vi "QBuf.vi"(3 "error in (no error)":errorcluster, 4 "pBufferHandle":i64, 5 "nInputHandle":u64) -> (0 "error out":errorcluster, 1 "GX_STATUS":i32, 2 "nOutputHandle":u64)   [LabVIEW 2016, in "GxLVLib.lvlib"]
uses:
  GxLVLib.lvlib
  GxIAPI.dll
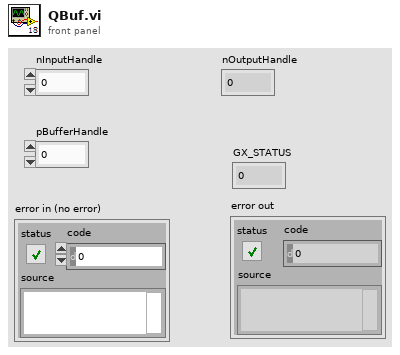
[diagram p1: front panel]
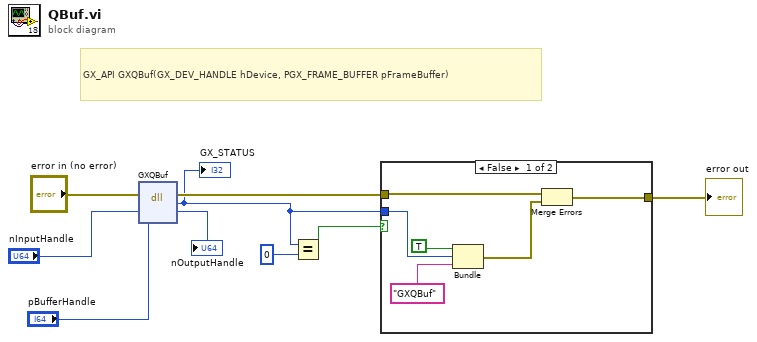
[diagram p0: block diagram]
diagram:
  # "GX_API GXQBuf(GX_DEV_HANDLE hDevice, PGX_FRAME_BUFFER pFrameBuffer)"
  n1 = dll-call lib="GxIAPI.dll" fn="GXQBuf"(error in="error in (no error)", "phDevice"="nInputHandle", "pBufferHandle"="pBufferHandle") -> (error out=w6:errorcluster, "GX_STATUS"=w3:i32, "phDevice"=→"nOutputHandle":i64)  [unwired: 3 in, 1 out]
  "GX_STATUS" <- w3
  n2 = Equal?(x=w3, y=0) -> (x = y?=w7:bool)
  n3 = case shown="False" w7 {
    tunnel: w6 -> [w15 w16]
    tunnel: [w14 w16] -> w5
    tunnel: w3 -> [w12 _]
    frame False {
      n4 = Bundle(TRUE, "GX_STATUS"=w12, "GXQBuf") -> (w13:cluster{bool, "GX_STATUS":i32, string})  [unwired: 1 in]
      n5 = Merge Errors(w15, w13) -> (w14:errorcluster)
    }
    frame True {
    }
  }
  "error out" <- w5
